vi "TestCounter.Get.vi"(8 "error in":errorcluster) -> (0 "error out":errorcluster, 2 "TestCount":u64, 5 "TestCount path":path)   [LabVIEW 2019, in "Tools.lvlib"]
uses:
  Tools.lvlib
  ProjectPaths.ctl
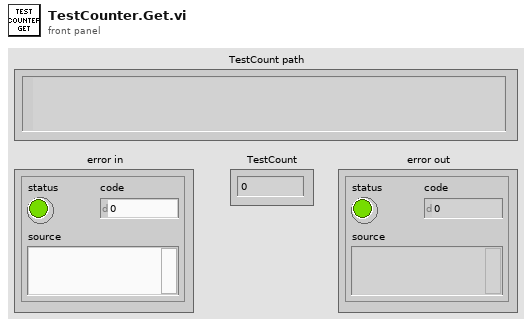
[diagram p1: front panel]
types:
  T1 = typedef "Tools.lvlib/ProjectPaths.ctl" = enum16{"Settings dir", "Logs dir", "Resources dir", "Verification file", "Users file", "Root dir"}
  T2 = enum16{"open", "replace", "create", "open or create", "replace or create", "replace or create with confirmation"}
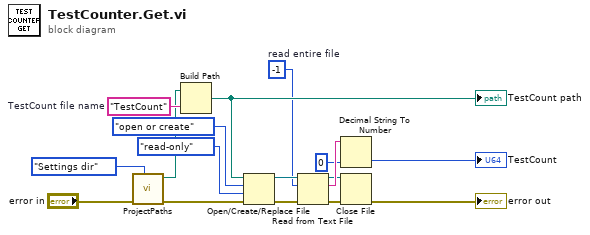
[diagram p0: block diagram]
diagram:
  w11 = -1  # read entire file
  w15 = "TestCount"  # TestCount file name
  n1 = call "ProjectPaths.vi"("Item"=ProjectPaths."Settings dir", "Error In"="error in") -> ("Error Out"=w3:errorcluster, "Path"=w2:path)  [unwired: 8 in]
  n2 = Build Path(base path=w2, name or relative path=w15) -> (appended path=w14:path)
  "TestCount path" <- w14
  n3 = Open/Create/Replace File(file path (use dialog)=w14, error in=w3, operation (0:open)=T2."open or create", access (0:read/write)=enum16{"read/write", "read-only", "write-only"}."read-only") -> (refnum out=w17:refnum<file>, error out=w16:errorcluster)  [unwired: 2 in, 1 out]
  n4 = Read from Text File(file (use dialog)=w17, count=w11, error in=w16) -> (refnum out=w6:refnum<file>, text=w10:string, error out=w5:errorcluster)  [unwired: 1 in, 1 out]
  n5 = Decimal String To Number(string=w10, default (0L)=u64 0 ("default (0 I32)")) -> (number=→"TestCount":u64)  [unwired: 1 in, 1 out]
  n6 = Close File(refnum=w6, error in=w5) -> (error out=→"error out":errorcluster)  [unwired: 1 out]
